vi "Assert Terminals.vi"(7 "Name":string="Undefined", 10 "Value in 2":variant, 11 "Value in 1":variant) -> (2 "Type Match":bool, 3 "Assertion Result":T1)   [LabVIEW 2020]
uses:
  Test Results.ctl
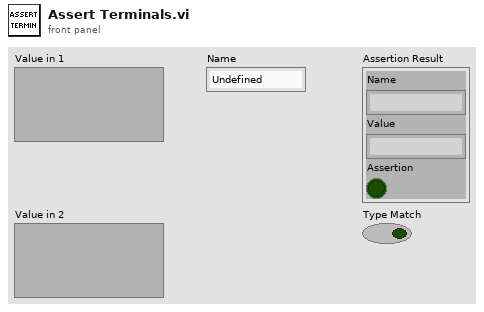
[diagram p1: front panel]
types:
  T1 = typedef "Test Results.ctl" = cluster{"Name":string, "Value":string, "Assertion":bool}
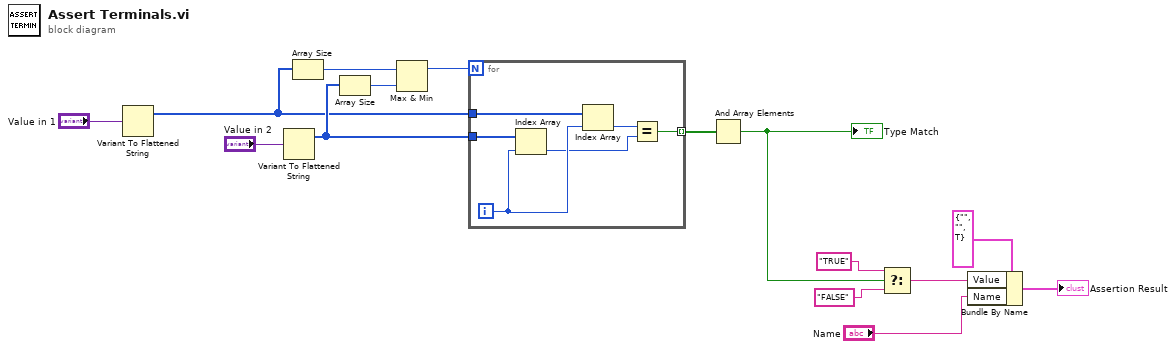
[diagram p0: block diagram]
diagram:
  n1 = Variant To Flattened String(Variant="Value in 1") -> (1:w11:i16[])  [unwired: 1 out]
  n2 = Variant To Flattened String(Variant="Value in 2") -> (1:w12:i16[])  [unwired: 1 out]
  n3 = Array Size(array=w11) -> (size(s)=w10:i32)
  n4 = Array Size(array=w12) -> (size(s)=w13:i32)
  n5 = Max & Min(x=w10, y=w13) -> (max(x,y)=w14:i32)  [unwired: 1 out]
  n6 = for {
    N: w14 -> [_]
    tunnel: w11 -> [w20]
    tunnel: w12 -> [w21]
    tunnel: [w16] -> w15 mode=indexing
    i -> [w19]
    n7 = Index Array(array=w21, index=w19) -> (element=w17:i16)
    n8 = Index Array(array=w20, index=w19) -> (element=w18:i16)
    n9 = Equal?(x=w18, y=w17) -> (x = y?=w16:bool)
  }
  n10 = And Array Elements(Boolean array=w15) -> (logical AND=w3:bool)
  "Type Match" <- w3
  n11 = Select(t="TRUE" ("Value"), s=w3, f="FALSE" ("Value")) -> (s? t:f=w7:string)
  n12 = Bundle By Name(cluster=T1 {"Name"="", "Value"="", "Assertion"=TRUE} ("Cluster"), "Value"=w7, "Name"="Name") -> (→"Assertion Result":T1)
